vi "SLL Check & Create Directory.vi"(8 "error in (no error)":errorcluster, 10 "Path is Directory? (F=No)":bool, 11 "Path":path) -> (0 "error out":errorcluster, 3 "Dup Path out":path)   [LabVIEW 2013]
doc: "This VI Check if thegiven directory(s) is available. if the directory is not available, then it creates those directories. If a file path is given it strips the filname and creates the directory.\n\nCopyright © 2006, Soliton Technologies. All rights reserved."
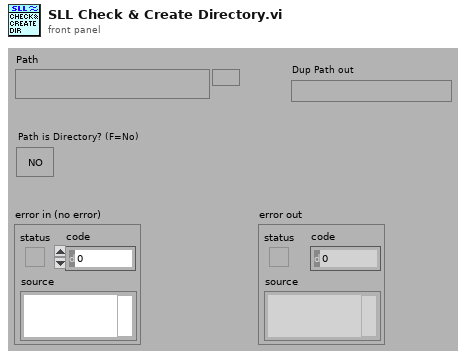
[diagram p1: front panel]
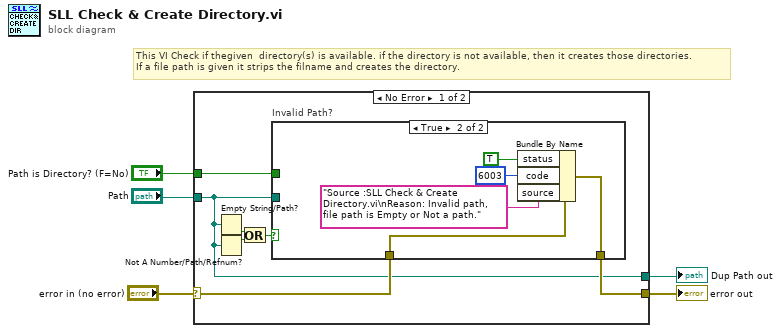
[diagram p0: block diagram]
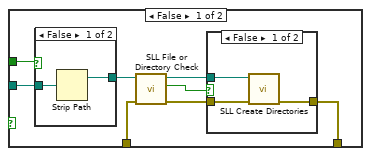
[diagram p2: hidden frame]
diagram:
  # "This VI Check if thegiven  directory(s) is available. if the directory is not available, then it creates those directories.\nIf a file path is given it strips the filname and creates the directory."
  n1 = case shown="No Error" "error in (no error)" {
    selector: "error in (no error)" -> [w11 w33]
    tunnel: "Path is Directory? (F=No)" -> [w12 _]
    tunnel: "Path" -> [w7 w34]
    tunnel: [w7 w34] -> w3
    tunnel: [w10 w33] -> w2
    frame No Error {
      n2 = Empty String/Path?(string/path=w7) -> (empty?=w8:bool)
      n3 = Not A Number/Path/Refnum?(number/path/refnum=w7) -> (NaN/Path/Refnum?=w9:bool)
      n4 = Or(x=w8, y=w9) -> (x .or. y?=w6:bool)
      n5 = case "Invalid Path?" shown="True" w6 {
        tunnel: w12 -> [w20 _]
        tunnel: w7 -> [w19 _]
        tunnel: w11 -> [w15 w29]
        tunnel: [w13 w28] -> w10
        frame False {
          n6 = case shown="False" w20 {
            tunnel: w19 -> [w26 w27]
            tunnel: [w25 w27] -> w16
            frame False {
              n7 = Strip Path(path=w26) -> (stripped path=w25:path)  [unwired: 1 out]
            }
            frame True {
            }
          }
          n8 = call "SLL File or Directory Check.vi"("error in (no error)"=w15, "File / directory path"=w16) -> ("error out"=w14:errorcluster, "exists?"=w17:bool, "dup file / directory path"=w18:path)  [unwired: 7 in]
          n9 = case shown="False" w17 {
            tunnel: w18 -> [w23 _]
            tunnel: w14 -> [w22 w24]
            tunnel: [w21 w24] -> w13
            frame False {
              n10 = call "SLL Create Directories.vi"("error in (no error)"=w22, "Filepath In"=w23) -> ("error out"=w21:errorcluster)  [unwired: 7 in, 2 out]
            }
            frame True {
            }
          }
        }
        frame True {
          n11 = Bundle By Name(cluster=w29, "status"=TRUE, "code"=6003, "source"="Source :SLL Check & Create Directory.vi\nReason: Invalid path, file path is Empty or Not a path.") -> (w28:errorcluster)
        }
      }
    }
    frame Error {
    }
  }
  "Dup Path out" <- w3
  "error out" <- w2
